vi "05a-multiple_functions.vi"() -> ()   [LabVIEW 2018, in "LV-0mq-Julia_roundtrip-lib.lvlib"]
uses:
  LV-0mq-Julia_roundtrip-lib.lvlib
  Server or client state.ctl
  detailed error info.ctl
  StackFrame.ctl
  Commands.ctl
  d2cb43a9-9305-42fb-ad58-bce983510195.vi
  d2cb43a9-9305-42fb-ad58-bce983510195.vi/e28c4e1c-617d-4a26-8291-f58a5accd33d.vi
  d2cb43a9-9305-42fb-ad58-bce983510195.vi/697b26af-9cff-4296-98ec-fa9d12ca8fdc.vi
  d2cb43a9-9305-42fb-ad58-bce983510195.vi/17159f77-75f5-4b7b-8d47-844af2eb1bcd.vi
  jl-scripts path.vi
  check ID validity.vi
  bindata_descr to JSON.vi
  check cluster field names.vi
  concat JSON.vi
panel:
  in  "operation":T1(radio)
  in  "operands":cluster{"x":dbl, "y":dbl}={"x"=2.0, "y"=2.0}
  in  "next":bool
  out "x+y":dbl=nan
  out "detailed error info":T2
  out "current error":errorcluster
  out "final error":errorcluster
  out "short err code":u8
  in  "stop":bool
  out "ZMQ timeout":bool
  out "Julia script file path":path
  out "temporary script path":path
  out "Jl Server state":T4
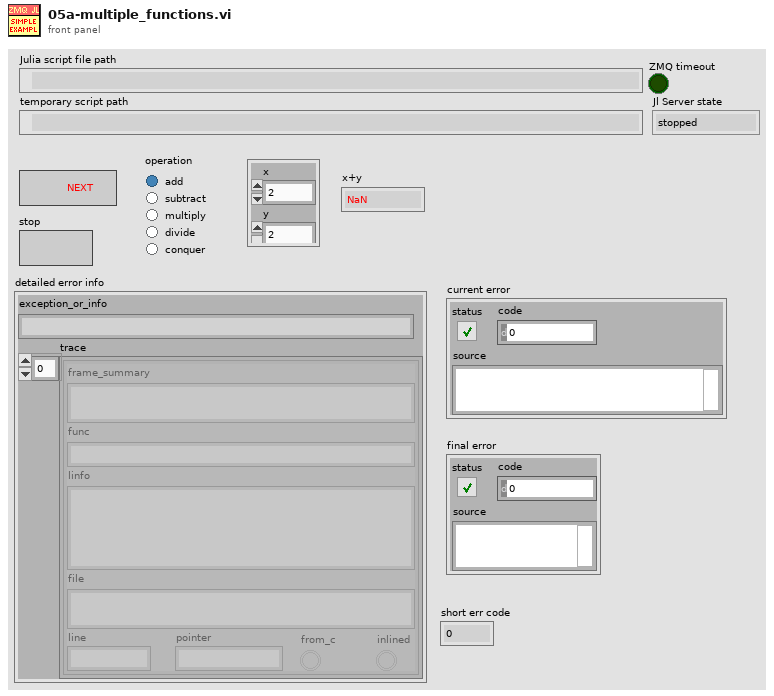
[diagram p1: front panel]
types:
  T1 = enum32{"add", "subtract", "multiply", "divide", "conquer"}
  T2 = typedef "LV-0mq-Julia_roundtrip-lib.lvlib/detailed error info.ctl" = cluster{"exception_or_info":string, "trace":T3[]}
  T3 = typedef "LV-0mq-Julia_roundtrip-lib.lvlib/StackFrame.ctl" = cluster{"frame_summary":string, "func":string, "linfo":string, "file":string, "line":i32, "pointer":u64, "from_c":bool, "inlined":bool}
  T4 = typedef "LV-0mq-Julia_roundtrip-lib.lvlib/Server or client state.ctl" = enum16{"stopped", "running", "unknown"}
  T5 = typedef "LV-0mq-Julia_roundtrip-lib.lvlib/Commands.ctl" = enum16{"Start Jl-server & Init LV-client", "Send request & Get response ", "Stop Jl-server & Cleanup LV-client", "Cleanup LV-client", "Start Jl-server", "Stop Jl-server", "Init LV-Client", "Cleanup LV-Client", "(not allowed)", "Set LV Client state", "Set Jl Server state", "set ZMQ timeout", "read ZMQ timeout", "read-out state"}
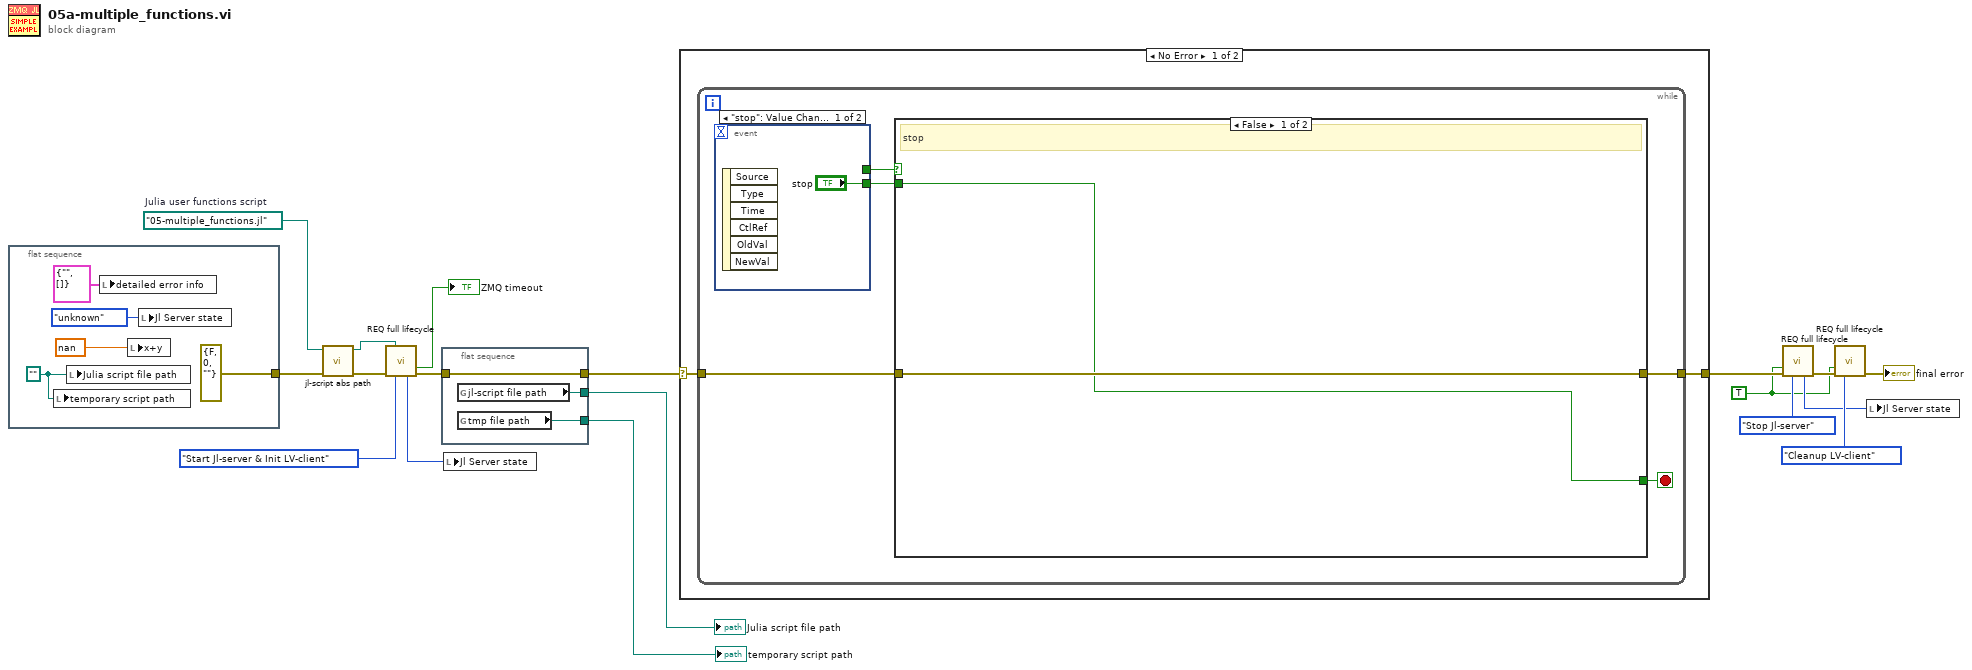
[diagram p0: block diagram]
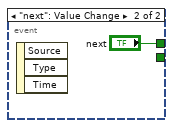
[diagram p2: hidden frame]
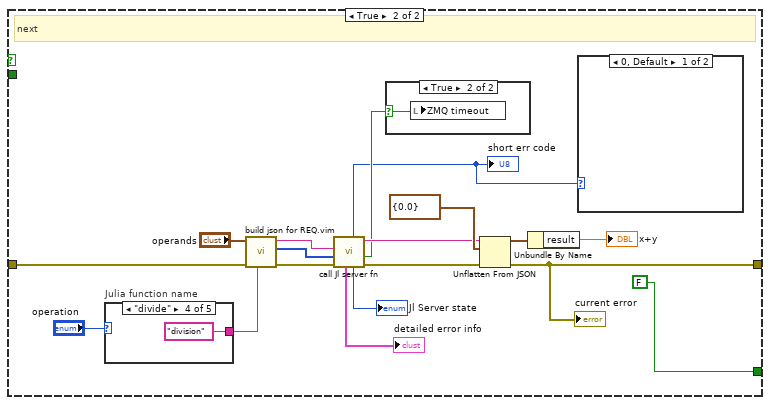
[diagram p3: hidden frame]
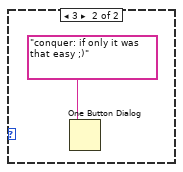
[diagram p4: hidden frame]
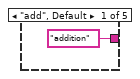
[diagram p5: hidden frame]
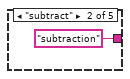
[diagram p6: hidden frame]
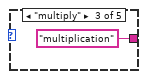
[diagram p7: hidden frame]
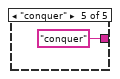
[diagram p8: hidden frame]
diagram:
  w4 = path "05-multiple_functions.jl"  # Julia user functions script
  w1 = TRUE ("Force command")
  n1 = flat-sequence {
    tunnel: [errorcluster {"status"=FALSE, "code"=0, "source"=""} ("error in (no error)")] -> w2
    frame #0 {
      w19 = path ""
      n2 = local write "temporary script path"(w19) -> ()
      n3 = local write "Julia script file path"(w19) -> ()
      n4 = local write "detailed error info"(T2 {"exception_or_info"="", "trace"=[]} ("detailed error info")) -> ()
      n5 = local write "x+y"(nan ("Server response")) -> ()
      n6 = local write "Jl Server state"(Server_or_client_state."unknown" ("Jl Server state out")) -> ()
    }
  }
  n7 = call "jl-script abs path.vi"("error in (no error)"=w2, "Julia user functions script"=w4) -> ("error out"=w5:errorcluster, "script abs path"=w6:path)  [unwired: 8 in]
  n8 = call "REQ full lifecycle.vi"("Julia user functions script"=w6, "error in"=w5, "command"=Commands."Start Jl-server & Init LV-client") -> ("timeout?"=→"ZMQ timeout":bool, "Jl Server state out"=w8:T4, "error out"=w7:errorcluster)  [unwired: 6 in, 4 out]
  n9 = flat-sequence {
    tunnel: [w26] -> w13
    tunnel: w7 -> [w26]
    tunnel: [w25] -> w11
    tunnel: [w24] -> w12
    frame #0 {
      n10 = global read "jl-scripts path.vi" "jl-script file path"() -> (w25:path)
      n11 = global read "jl-scripts path.vi" "tmp file path"() -> (w24:path)
    }
  }
  n12 = local write "Jl Server state"(w8) -> ()
  n13 = case shown="No Error" w13 {
    selector: w13 -> [w27 w63]
    tunnel: [w28 w63] -> w18
    frame No Error {
      n14 = while {
        tunnel: w27 -> [w32]
        tunnel: [w33] -> w28
        stop <- w30 stop-if-true
        n15 = event shown="[0] \"stop\": Value Change" {
          selector: _ -> [_ _]
          dyn-events: _ -> [_ _]
          timeout: _ -> [_ _]
          tunnel: [_ "next"] -> w31
          tunnel: ["stop" _] -> w29
          event "stop": Value Change {
            n16 = event-data() -> ()  [unwired: 1 in, 6 out]
          }
          event "next": Value Change {
            n17 = event-data() -> ()  [unwired: 1 in, 3 out]
          }
        }
        n18 = case shown="False" w31 {
          tunnel: [w37 w51] -> w33
          tunnel: w32 -> [w37 w53]
          tunnel: [w36 FALSE ("stop this VI only")] -> w30
          tunnel: w29 -> [w36 _]
          frame False {
            # "stop"
          }
          frame True {
            # "next"
            n19 = case "Julia function name" shown="\"divide\"" "operation" {
              tunnel: ["addition" "subtraction" "multiplication" "division" "conquer"] -> w39
              frame "add", Default {
              }
              frame "subtract" {
              }
              frame "multiply" {
              }
              frame "divide" {
              }
              frame "conquer" {
              }
            }
            n20 = call "build json for REQ.vim"("fun2call"=w39, "error in (no error)"=w53, "Arguments 1"="operands") -> ("error out"=w47:errorcluster, "bindata out"=w48:u8[], "JSON string out"=w49:string)  [unwired: 6 in]
            n21 = call "call Jl server fn.vi"("error in (no error)"=w47, "binary data in"=w48, "JSON string in"=w49) -> ("error out"=w43:errorcluster, "timeout?"=w41:bool, "JSON received"=w45:string, "Jl Server state out"=→"Jl Server state":T4, "return code"=w38:u8, "detailed error info"=→"detailed error info":T2)  [unwired: 2 in, 1 out]
            "short err code" <- w38
            n22 = case shown="True" w41 {
              selector: w41 -> [_ w62]
              frame False {
              }
              frame True {
                n23 = local write "ZMQ timeout"(w62) -> ()
              }
            }
            n24 = Unflatten From JSON(JSON string=w45, type and defaults=cluster{"result":dbl} {"result"=0.0} ("parsed response"), error in (no error)=w43) -> (value=w54:cluster{"result":dbl}, error out=w51:errorcluster)  [unwired: 4 in]
            "current error" <- w51
            n25 = Unbundle By Name(w54) -> ("result"=→"x+y":dbl)
            n26 = case shown="0, Default" w38 {
              frame 0, Default {
              }
              frame 3 {
                n27 = One Button Dialog(message="conquer: if only it was that easy ;)") -> ()  [unwired: 1 in, 1 out]
              }
            }
          }
        }
      }
    }
    frame Error {
    }
  }
  n28 = call "REQ full lifecycle.vi"("Force command"=w1, "error in"=w18, "command"=Commands."Stop Jl-server") -> ("Jl Server state out"=w10:T4, "error out"=w16:errorcluster)  [unwired: 6 in, 5 out]
  n29 = call "REQ full lifecycle.vi"("Force command"=w1, "error in"=w16, "command"=Commands."Cleanup LV-client") -> ("error out"=→"final error":errorcluster)  [unwired: 6 in, 6 out]
  n30 = local write "Jl Server state"(w10) -> ()
  "temporary script path" <- w12
  "Julia script file path" <- w11
